vi "TestPDO.vi"() -> ()   [LabVIEW 2017]
uses:
  Orion_BMS.lvclass
  <vilib>/userdefined/High Color/nirio_resource_hc.ctl
  TypeDef_BMSData.ctl
  TypeDef_BmsStatus.ctl
  Orion_BMS.lvclass/Orion_BMS.ctl
  <vilib>/FPGAPlugInAG/cRIO-9063/niLvFpga_Open_cRIO-9063.vi
  <vilib>/rvi/interface/common/dynamic/niFpgaDynamicAddResources.vi
  <vilib>/FPGAPlugInAG/Dynamic/niLvFpga_Close_Dynamic.vi
  <vilib>/rvi/interface/nirviOpenFPGA/nirviOpenFPGA.xnode
  FPGA Bitfiles/TheMacroProject_FPGATarget_Fail-SafeControl_eeRwxioMFzY.lvbitx
  <vilib>/rvi/interface/nirviCloseFPGA/nirviCloseFPGA.xnode
panel:
  out "ChecksumMatched":bool
  out "BMS Data":T1
  out "LoopCount":i32
  in  "resource name":T3
  in  "stop":bool
  in  "PDO channel":u8(ring) items=["PDO 1", "PDO 2", "PDO 3", "PDO 4"]
  out "error out":errorcluster
  in  "error in (no error)":errorcluster
  in  "Orion_BMS.lvclass":refnum<class "Orion_BMS.lvclass">
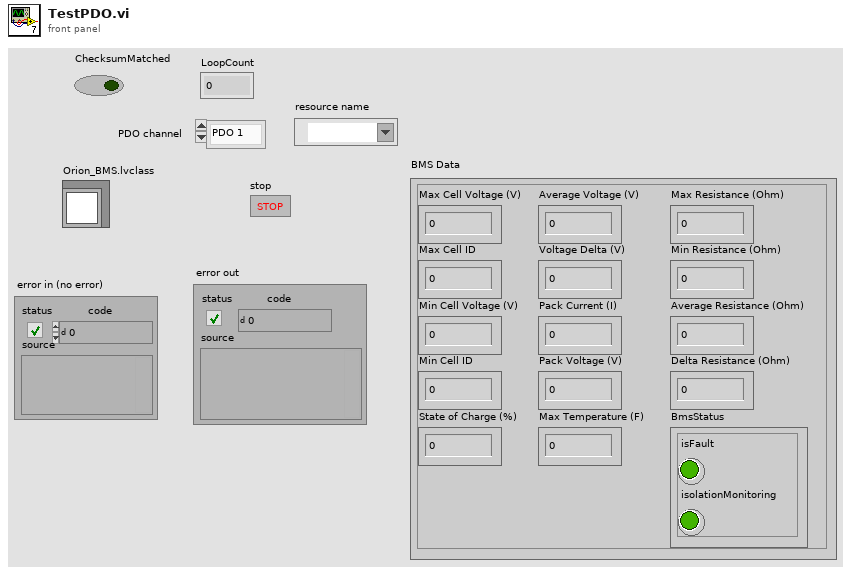
[diagram p1: front panel]
types:
  T1 = typedef "TypeDef_BMSData.ctl" = cluster{"Max Cell Voltage (V)":dbl, "Max Cell ID":dbl, "Min Cell Voltage (V)":dbl, "Min Cell ID":dbl, "State of Charge (%)":dbl, "Average Voltage (V)":dbl, "Voltage Delta (V)":dbl, "Pack Current (I)":dbl, "Pack Voltage (V)":dbl, "Max Resistance (Ohm)":dbl, "Min Resistance (Ohm)":dbl, "Average Resistance (Ohm)":dbl, "Delta Resistance (Ohm)":dbl, "BmsStatus":T2, "Max Temperature (F)":dbl}
  T2 = typedef "TypeDef_BmsStatus.ctl" = cluster{"isFault":bool, "isolationMonitoring":bool}
  T3 = typedef "nirio_resource_hc.ctl" = tag
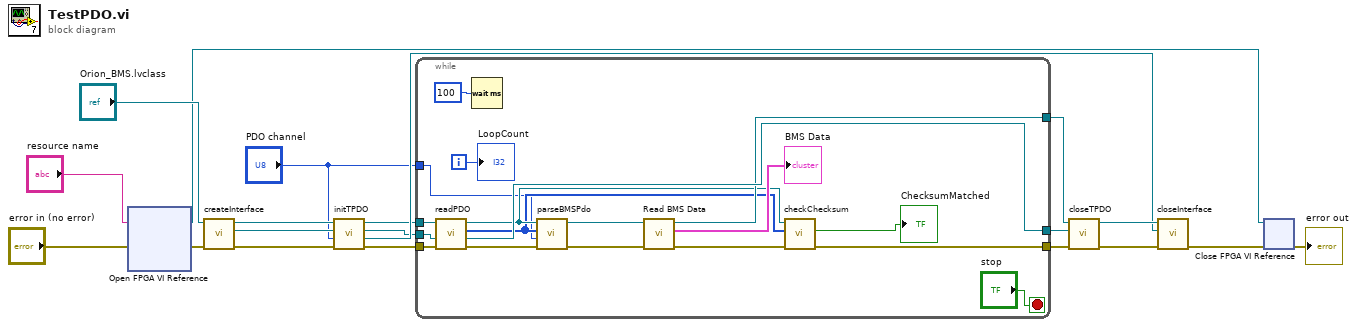
[diagram p0: block diagram]
diagram:
  n1 = xnode "Open FPGA VI Reference"("error in"="error in (no error)", "resource name"="resource name") -> ("FPGA VI Reference Out"=w4:refnum<k20>, "error out"=w7:errorcluster)
  n2 = call "createInterface.vi"("error in (no error)"=w7, "Orion_BMS in"="Orion_BMS.lvclass") -> ("error out"=w14:errorcluster, "interface object out"=w17:refnum<k20>, "Orion_BMS out"=w16:refnum<class "Orion_BMS.lvclass">)  [unwired: 7 in]
  n3 = call "initTPDO.vi"("error in (no error)"=w14, "PDO channel"="PDO channel", "interface object in"=w17, "Orion_BMS in"=w16) -> ("error out"=w12:errorcluster, "interface object out"=w15:refnum<k20>, "TPDO object out"=w11:refnum<k20>, "Orion_BMS out"=w13:refnum<class "Orion_BMS.lvclass">)  [unwired: 4 in]
  n4 = while {
    tunnel: w12 -> [w38]
    tunnel: w13 -> [w37]
    tunnel: w11 -> [w36]
    tunnel: [w35] -> w10
    tunnel: "PDO channel" -> [w24]
    tunnel: [w22] -> w2
    tunnel: [w28] -> w1
    i -> [w33]
    stop <- "stop" stop-if-true
    n5 = call "readPDO.vi"("error in (no error)"=w38, "TPDO object in"=w36, "Orion_BMS in"=w37) -> ("error out"=w26:errorcluster, "TPDO object out"=w35:refnum<k20>, "TPDO data"=w25:u8[], "Orion_BMS out"=w27:refnum<class "Orion_BMS.lvclass">)  [unwired: 4 in, 1 out]
    n6 = Wait (ms)(milliseconds to wait=u32 100) -> ()  [unwired: 1 out]
    n7 = call "parseBMSPdo.vi"("error in (no error)"=w26, "PDO channel"=w24, "TPDO data"=w25, "Orion_BMS in"=w27) -> ("error out"=w30:errorcluster, "Orion_BMS out"=w31:refnum<class "Orion_BMS.lvclass">)  [unwired: 6 in]
    n8 = call "Read BMS Data.vi"("error in (no error)"=w30, "Orion_BMS in"=w31) -> ("error out"=w23:errorcluster, "BMS Data"=→"BMS Data":T1, "Orion_BMS out"=w28:refnum<class "Orion_BMS.lvclass">)  [unwired: 7 in]
    n9 = call "checkChecksum.vi"("error in (no error)"=w23, "TPDO data"=w25, "Orion_BMS in"=w27) -> ("error out"=w22:errorcluster, "checkSumMatched"=→"ChecksumMatched":bool)  [unwired: 6 in, 1 out]
    "LoopCount" <- w33
  }
  n10 = call "closeTPDO.vi"("error in (no error)"=w2, "TPDO object in"=w10, "Orion_BMS in"=w1) -> ("error out"=w18:errorcluster, "Orion_BMS out"=w19:refnum<class "Orion_BMS.lvclass">)  [unwired: 7 in]
  n11 = call "closeInterface.vi"("error in (no error)"=w18, "interface object in"=w15, "Orion_BMS in"=w19) -> ("error out"=w6:errorcluster)  [unwired: 7 in, 1 out]
  n12 = xnode "Close FPGA VI Reference"("FPGA VI Reference In"=w4, "error in"=w6) -> ("error out"=→"error out":errorcluster)
